vi "Close.vi"(8 "error in (no error)":errorcluster, 11 "Multi Column Listbox in":refnum<class "Multi Column Listbox.lvclass">) -> (0 "error out":errorcluster, 3 "Multi Column Listbox out":refnum<class "Multi Column Listbox.lvclass">)   [LabVIEW 2013, in "Table Manager.lvlib" / "Multi Column Listbox.lvclass"]
uses:
  Multi Column Listbox.lvclass
  Table Manager/Table Manager.lvclass
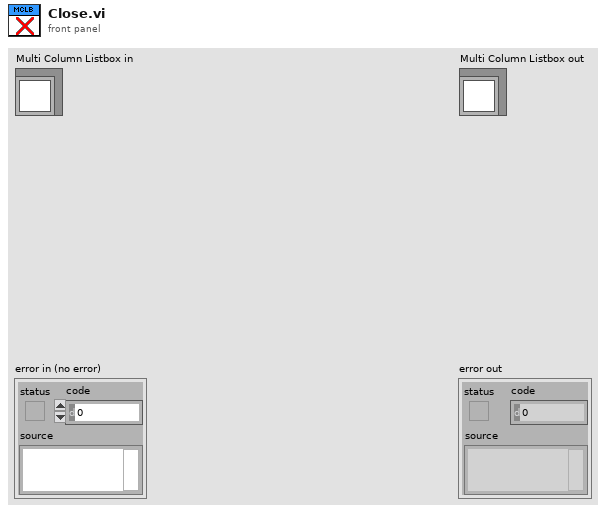
[diagram p1: front panel]
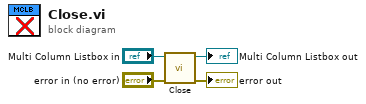
[diagram p0: block diagram]
diagram:
  n1 = call-parent "Close.vi"("error in (no error)"="error in (no error)", "table manager in"="Multi Column Listbox in") -> ("error out"=→"error out":errorcluster, "table manager out"=→"Multi Column Listbox out":refnum<class "Multi Column Listbox.lvclass">)  [unwired: 8 in]
